vi "Write Armed.vi"(8 "error in (no error)":errorcluster, 10 "Armed":bool, 11 "Pulse Recorder in":refnum<class "Pulse Recorder Actor.lvclass">) -> (0 "error out":errorcluster, 3 "Pulse Recorder out":refnum<class "Pulse Recorder Actor.lvclass">)   [LabVIEW 2021, in "Pulse Recorder Actor.lvclass"]
uses:
  Pulse Recorder Actor.lvclass
  Pulse Recorder Actor.lvclass/Pulse Recorder Actor.ctl
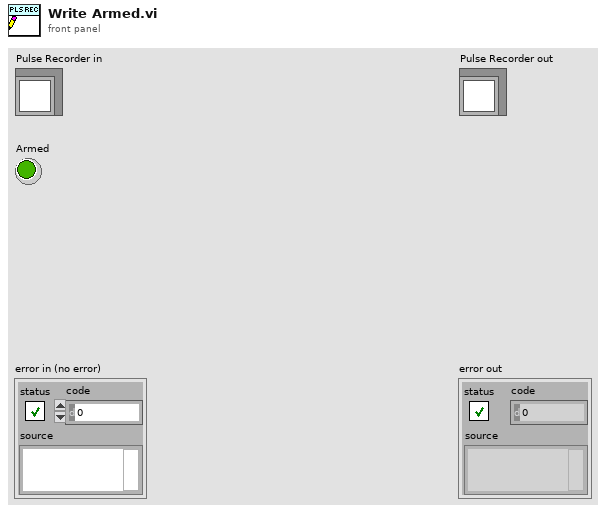
[diagram p1: front panel]
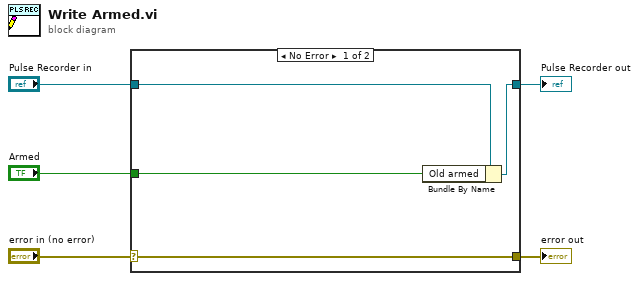
[diagram p0: block diagram]
diagram:
  n1 = case shown="No Error" "error in (no error)" {
    selector: "error in (no error)" -> [w9 w10]
    tunnel: [w9 w10] -> w4
    tunnel: [w7 w11] -> w2
    tunnel: "Pulse Recorder in" -> [w8 w11]
    tunnel: "Armed" -> [w6 _]
    frame No Error {
      n2 = Bundle By Name(cluster=w8, "Old armed"=w6) -> (w7:refnum<class "Pulse Recorder Actor.lvclass">)
    }
    frame Error {
    }
  }
  "error out" <- w4
  "Pulse Recorder out" <- w2
